vi "MOTOR SEQUENCE.vi"() -> ()   [LabVIEW 2019]
uses:
  <vilib>/MakerHub/LINX/Public/Peripherals/Digital/Digital Write 1 Chan.vi
  <vilib>/MakerHub/LINX/Public/Peripherals/PWM/PWM Set Duty Cycle 1 Chan.vi
  <vilib>/MakerHub/LINX/Public/Peripherals/Digital/Digital Write N Chans.vi
  <vilib>/MakerHub/LINX/Private/Local IO/LinxDigitalWrite.vi
  <vilib>/MakerHub/LINX/Public/Utilities/Check Channel.vi
  <vilib>/MakerHub/LINX/Public/Utilities/Open Serial.vi
  <vilib>/MakerHub/LINX/Private/Utilties/Generate Error.vi
  <vilib>/MakerHub/LINX/Public/Peripherals/PWM/PWM Set Duty Cycle N Chans.vi
  <vilib>/MakerHub/LINX/LMH-LINX.lvlib
panel:
  in  "Serial Port":refnum<visa-resource-name>="N/A"
  in  "PWM Channel":u8
  in  "DO Channel 2":u8
  in  "DO Channel":u8
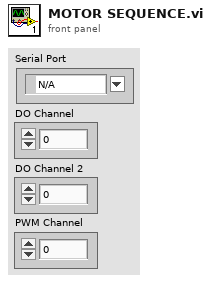
[diagram p1: front panel]
types:
  T1 = typedef "LMH-LINX.lvlib/LINX Ref.ctl" = cluster{"IO":T2, "Interface":T3, "LINX Device Config":T4}
  T2 = typedef "LMH-LINX.lvlib/Platform.ctl" = enum16{"Remote", "Local"}
  T3 = typedef "LMH-LINX.lvlib/Interface.ctl" = enum16{"Serial", "TCP"}
  T4 = typedef "LMH-LINX.lvlib/Device.lvlib/LINX Device Config.ctl" = cluster{"Interface":T3, "COM Port":refnum<visa-resource-name>, "TCP Configuration":T5, "Device Family":u8, "Device ID":u8, "Device Name":string, "TCP Ref":refnum<k5>, "Channels":T6}
  T5 = typedef "LMH-LINX.lvlib/Device.lvlib/TCP Config.ctl" = cluster{"IP Address":string, "Port":u16}
  T6 = typedef "LMH-LINX.lvlib/Channels.ctl" = cluster{"DI":u8[], "DO":u8[], "AI":u8[], "AO":u8[], "PWM":u8[], "QE":u8[], "UART":u8[], "I2C 2":u8[], "SPI":u8[], "CAN":u8[], "Servo":u8[], "AI Ref (V)":dbl, "AI Resolution (Bits)":u8, "AO Ref (V)":dbl, "AO Resolution (Bits)":u8}
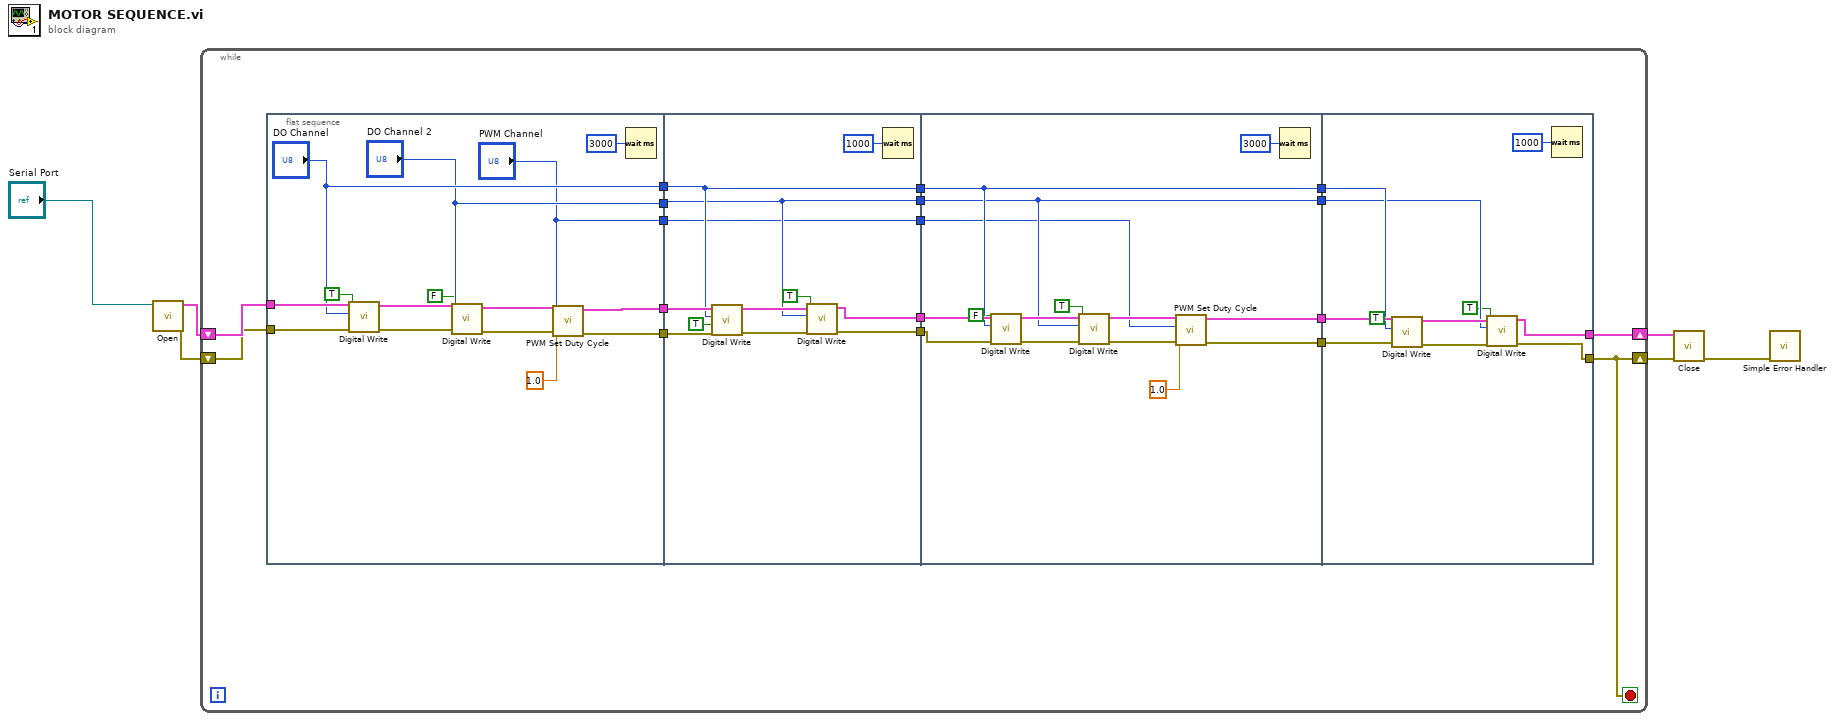
[diagram p0: block diagram]
diagram:
  n1 = call-poly <vilib>:"Open.vi"("Serial Port"="Serial Port") -> ("Error Out"=w4:errorcluster, "LINX Resource"=w6:T1)  [unwired: 8 in, 1 out]
  n2 = while {
    shift-right: [w9] -> w5
    shift-left: w6 -> [w10]
    shift-right: [w7] -> w3
    shift-left: w4 -> [w8]
    stop <- w7 stop-if-true
    n3 = flat-sequence {
      tunnel: w10 -> [w39]
      tunnel: [w36] -> w24
      tunnel: [w33] -> w23
      tunnel: w8 -> [w32]
      tunnel: ["DO Channel"] -> w22
      tunnel: ["DO Channel 2"] -> w21
      tunnel: ["PWM Channel"] -> w20
      tunnel: w24 -> [w51]
      tunnel: [w49] -> w19
      tunnel: w23 -> [w48]
      tunnel: [w46] -> w18
      tunnel: w22 -> [w45]
      tunnel: [w45] -> w17
      tunnel: w21 -> [w44]
      tunnel: [w44] -> w16
      tunnel: w20 -> [w43]
      tunnel: [w43] -> w15
      tunnel: w19 -> [w66]
      tunnel: [w63] -> w14
      tunnel: w18 -> [w62]
      tunnel: [w59] -> w13
      tunnel: w17 -> [w58]
      tunnel: [w58] -> w12
      tunnel: w16 -> [w57]
      tunnel: [w57] -> w11
      tunnel: w15 -> [w56]
      tunnel: w14 -> [w77]
      tunnel: [w75] -> w9
      tunnel: w13 -> [w74]
      tunnel: [w72] -> w7
      tunnel: w12 -> [w71]
      tunnel: w11 -> [w70]
      frame #0 {
        n4 = call-poly <vilib>:"Digital Write.vi"("Error In"=w32, "Output Value"=TRUE, "DO Channel"="DO Channel", "LINX Resource"=w39) -> ("Error Out"=w35:errorcluster, "LINX Resource"=w38:T1)  [unwired: 6 in]
        n5 = call-poly <vilib>:"Digital Write.vi"("Error In"=w35, "Output Value"=FALSE, "DO Channel"="DO Channel 2", "LINX Resource"=w38) -> ("Error Out"=w34:errorcluster, "LINX Resource"=w37:T1)  [unwired: 6 in]
        n6 = call-poly <vilib>:"PWM Set Duty Cycle.vi"("Error In"=w34, "Duty Cycle (0-1)"=1.0, "PWM Channel"="PWM Channel", "LINX Resource"=w37) -> ("Error Out"=w33:errorcluster, "LINX Resource"=w36:T1)  [unwired: 6 in]
        n7 = Wait (ms)(milliseconds to wait=u32 3000) -> ()  [unwired: 1 out]
      }
      frame #1 {
        n8 = call-poly <vilib>:"Digital Write.vi"("Error In"=w48, "Output Value"=TRUE, "DO Channel"=w45, "LINX Resource"=w51) -> ("Error Out"=w47:errorcluster, "LINX Resource"=w50:T1)  [unwired: 6 in]
        n9 = call-poly <vilib>:"Digital Write.vi"("Error In"=w47, "Output Value"=TRUE, "DO Channel"=w44, "LINX Resource"=w50) -> ("Error Out"=w46:errorcluster, "LINX Resource"=w49:T1)  [unwired: 6 in]
        n10 = Wait (ms)(milliseconds to wait=u32 1000) -> ()  [unwired: 1 out]
      }
      frame #2 {
        n11 = call-poly <vilib>:"Digital Write.vi"("Error In"=w62, "Output Value"=FALSE, "DO Channel"=w58, "LINX Resource"=w66) -> ("Error Out"=w61:errorcluster, "LINX Resource"=w65:T1)  [unwired: 6 in]
        n12 = call-poly <vilib>:"Digital Write.vi"("Error In"=w61, "Output Value"=TRUE, "DO Channel"=w57, "LINX Resource"=w65) -> ("Error Out"=w60:errorcluster, "LINX Resource"=w64:T1)  [unwired: 6 in]
        n13 = call-poly <vilib>:"PWM Set Duty Cycle.vi"("Error In"=w60, "Duty Cycle (0-1)"=1.0, "PWM Channel"=w56, "LINX Resource"=w64) -> ("Error Out"=w59:errorcluster, "LINX Resource"=w63:T1)  [unwired: 6 in]
        n14 = Wait (ms)(milliseconds to wait=u32 3000) -> ()  [unwired: 1 out]
      }
      frame #3 {
        n15 = call-poly <vilib>:"Digital Write.vi"("Error In"=w74, "Output Value"=TRUE, "DO Channel"=w71, "LINX Resource"=w77) -> ("Error Out"=w73:errorcluster, "LINX Resource"=w76:T1)  [unwired: 6 in]
        n16 = call-poly <vilib>:"Digital Write.vi"("Error In"=w73, "Output Value"=TRUE, "DO Channel"=w70, "LINX Resource"=w76) -> ("Error Out"=w72:errorcluster, "LINX Resource"=w75:T1)  [unwired: 6 in]
        n17 = Wait (ms)(milliseconds to wait=u32 1000) -> ()  [unwired: 1 out]
      }
    }
  }
  n18 = call <vilib>:"Close.vi"("Error In"=w3, "LINX Resource"=w5) -> ("Error Out"=w2:errorcluster)  [unwired: 9 in]
  n19 = call <vilib>:"Simple Error Handler.vi"("error in (no error)"=w2) -> ()  [unwired: 4 in, 5 out]
